vi "Testing Utility.vi"() -> ()   [LabVIEW 2009]
uses:
  <vilib>/Analysis/NI_AALPro.lvlib
panel:
  out "x-y":u32
  in  "Prediction Time":dbl
  out "XY Graph 2":cluster{dbl[], dbl[]}(graph)
  out "XY Graph":cluster{dbl[], dbl[]}(graph)
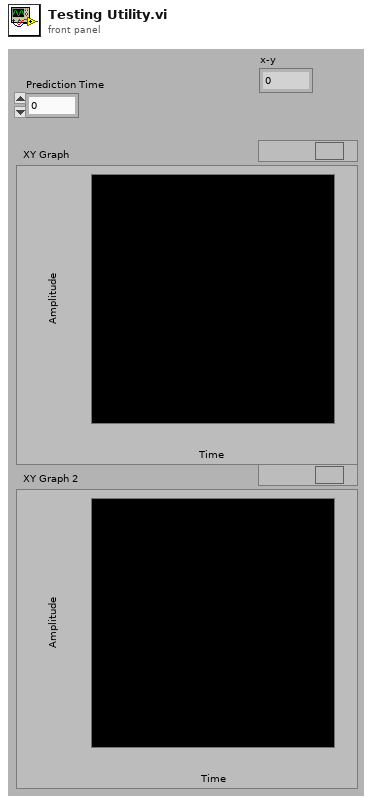
[diagram p1: front panel]
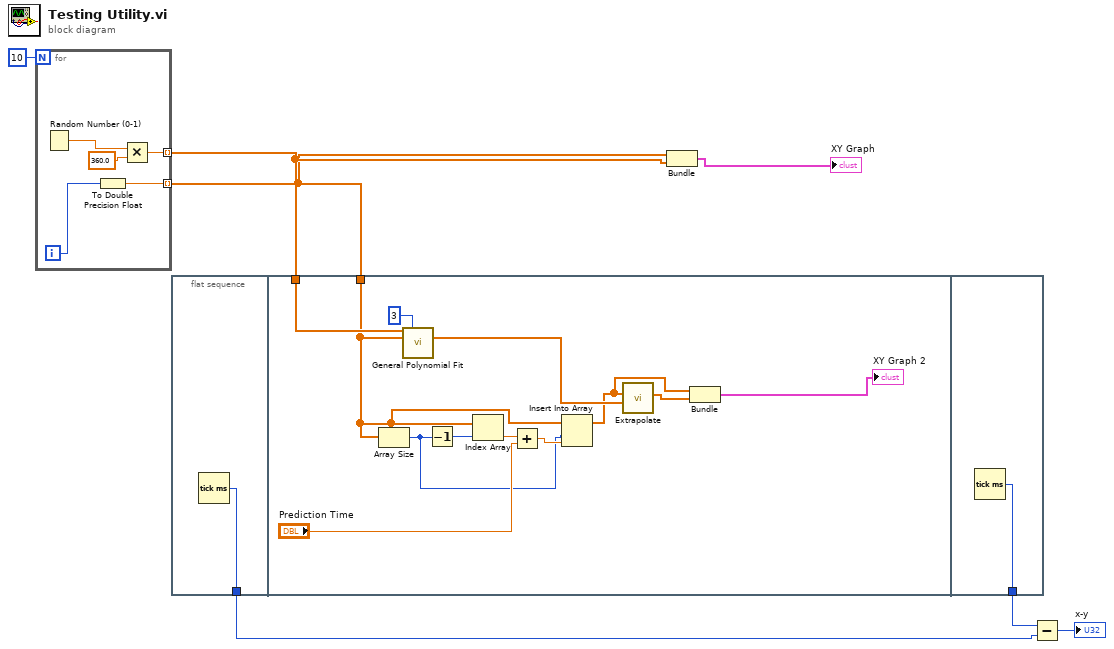
[diagram p0: block diagram]
diagram:
  n1 = for {
    N: 10 -> [_]
    tunnel: [w9] -> w5 mode=indexing
    tunnel: [w10] -> w4 mode=indexing
    i -> [w11]
    n2 = Random Number (0-1)() -> (number: 0 to 1=w12:dbl)
    n3 = To Double Precision Float(number=w11) -> (double precision float=w10:dbl)
    n4 = Multiply(x=w12, y=360.0) -> (x*y=w9:dbl)
  }
  n5 = flat-sequence {
    tunnel: [w13] -> w2
    tunnel: w5 -> [w21]
    tunnel: w4 -> [w15]
    tunnel: [w26] -> w3
    frame #0 {
      n6 = Tick Count (ms)() -> (millisecond timer value=w13:u32)
    }
    frame #1 {
      n7 = Array Size(array=w15) -> (size(s)=w17:i32)
      n8 = call <vilib>:"General Polynomial Fit.vi"("Y"=w21, "polynomial order"=3, "X"=w15) -> ("Polynomial Coefficients"=w24:dbl[])  [unwired: 9 in, 3 out]
      n9 = Decrement(x=w17) -> (x-1=w14:i32)
      n10 = Index Array(array=w15, index=w14) -> (element=w20:dbl)
      n11 = Add(x=w20, y="Prediction Time") -> (x+y=w18:dbl)
      n12 = Insert Into Array(array=w15, index=w17, new element=w18) -> (w16:dbl[])
      n13 = call "Extrapolate.vi"("Polynomial Coefficients"=w24, "xi"=w16) -> ("yi"=w23:dbl[])  [unwired: 9 in]
      n14 = Bundle(w16, "yi"=w23) -> (→"XY Graph 2":cluster{dbl[], "yi":dbl[]})  [unwired: 1 in]
    }
    frame #2 {
      n15 = Tick Count (ms)() -> (millisecond timer value=w26:u32)
    }
  }
  n16 = Bundle(w4, w5) -> (→"XY Graph":cluster{dbl[], dbl[]})  [unwired: 1 in]
  n17 = Subtract(x=w3, y=w2) -> (x-y=→"x-y":u32)
